vi "GetFault_PIGEON2_BootupAccel.vi"(9 "timeoutSeconds":dbl, 10 "WaitForUpdate":bool=TRUE, 11 "DeviceReference":T2) -> (3 "Output":T1)   [LabVIEW 2023]
uses:
  Users/Cory/Documents/PhoenixPro-LabVIEW-Generation/controls/DeviceReference.ctl
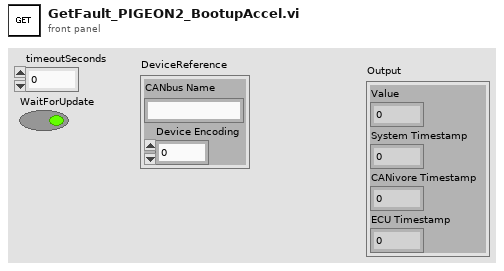
[diagram p1: front panel]
types:
  T1 = cluster{"Value":dbl, "System Timestamp":dbl, "CANivore Timestamp":dbl, "ECU Timestamp":dbl}
  T2 = typedef "DeviceReference.ctl" = cluster{"CANbus Name":string, "Device Encoding":u32}
  T3 = cluster{"OutValue":dbl, "Units":cluster{"Numeric":u8, "Numeric 2":u8, "Numeric 3":u8, "Numeric 4":u8, "Numeric 5":u8, "Numeric 6":u8, "Numeric 7":u8, "Numeric 8":u8, "Numeric 9":u8, "Numeric 10":u8}, "swTimestampSeconds":dbl, "hwTimestampSeconds":dbl, "ecuTimestampSeconds":dbl, "error":i32}
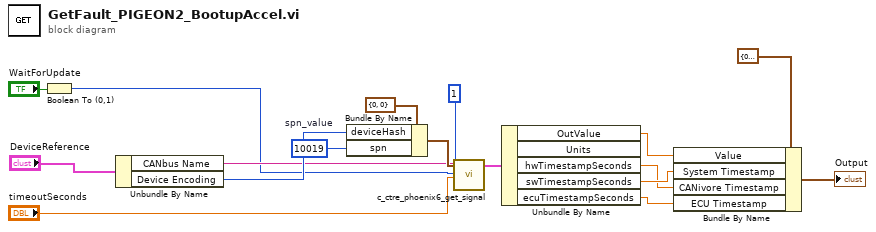
[diagram p0: block diagram]
diagram:
  w10 = u32 10019  # spn_value
  n1 = Boolean To (0,1)(Boolean="WaitForUpdate") -> (0, 1=w2:i16)
  n2 = Unbundle By Name("DeviceReference") -> ("CANbus Name"=w3:string, "Device Encoding"=w11:u32)
  n3 = Bundle By Name(cluster=cluster{"deviceHash":u32, "spn":u32} {"deviceHash"=0, "spn"=0} ("Cluster"), "deviceHash"=w11, "spn"=w10) -> (w12:cluster{"deviceHash":u32, "spn":u32})
  n4 = call <vilib>:"c_ctre_phoenix6_get_signal.vi"("Numeric 2"=u32 1 ("num_signals"), "Cluster"=w12, "String 2"=w3, "Numeric 3"=w2, "Numeric 4"="timeoutSeconds") -> ("Cluster 2"=w8:T3)  [unwired: 20 in, 2 out]
  n5 = Unbundle By Name(w8) -> ("OutValue"=w7:dbl, "hwTimestampSeconds"=w5:dbl, "swTimestampSeconds"=w6:dbl, "ecuTimestampSeconds"=w4:dbl)  [unwired: 1 out]
  n6 = Bundle By Name(cluster=T1 {"Value"=0.0, "System Timestamp"=0.0, "CANivore Timestamp"=0.0, "ECU Timestamp"=0.0} ("Output 2"), "Value"=w7, "System Timestamp"=w6, "CANivore Timestamp"=w5, "ECU Timestamp"=w4) -> (→"Output":T1)
